vi "StartCapture.vi"(8 "error in (no error)":errorcluster, 10 "Continuous":bool, 11 "ImagingDevice in":refnum<class "ImagingDevice.lvclass">) -> (0 "error out":errorcluster, 3 "ImagingDevice out":refnum<class "ImagingDevice.lvclass">)   [LabVIEW 2023, in "ImagingDevice.lvclass"]
uses:
  ImagingDevice.lvclass
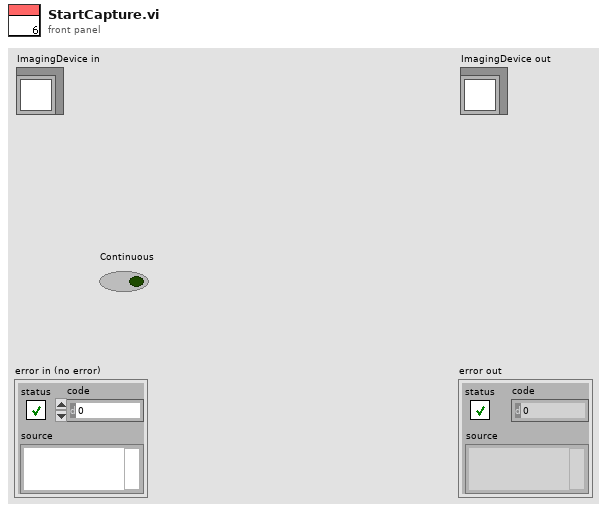
[diagram p1: front panel]
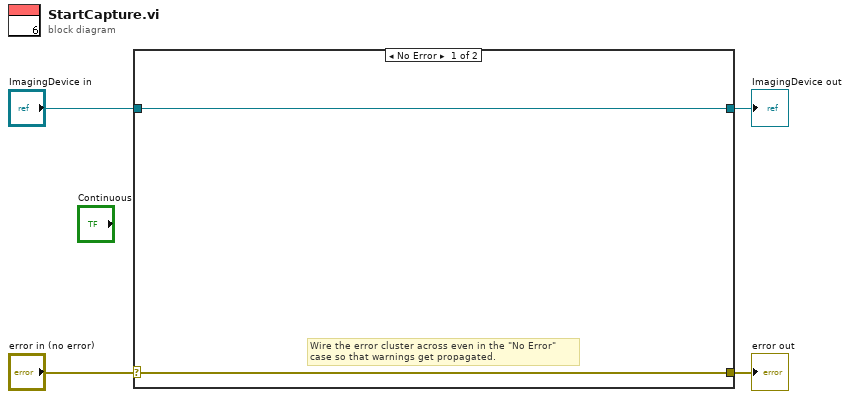
[diagram p0: block diagram]
diagram:
  n1 = case shown="No Error" "error in (no error)" {
    selector: "error in (no error)" -> [w5 w8]
    tunnel: [w5 w8] -> w3
    tunnel: [w6 w7] -> w1
    tunnel: "ImagingDevice in" -> [w6 w7]
    frame No Error {
      # "Wire the error cluster across even in the \"No Error\"\ncase so that warnings get propagated."
    }
    frame Error {
    }
  }
  "error out" <- w3
  "ImagingDevice out" <- w1
